vi "target.set.vi"(8 "error in (no error)":errorcluster, 10 "datasources.lvlib:target.lvclass":refnum<class "target.lvclass">, 11 "datasource in":refnum<class "datasource.lvclass">) -> (0 "error out":errorcluster, 3 "datasource out":refnum<class "datasource.lvclass">)   [LabVIEW 2020, in "datasources.lvlib" / "datasource.lvclass"]
uses:
  datasource.lvclass
  target/target.lvclass
  datasource.lvclass/datasource.ctl
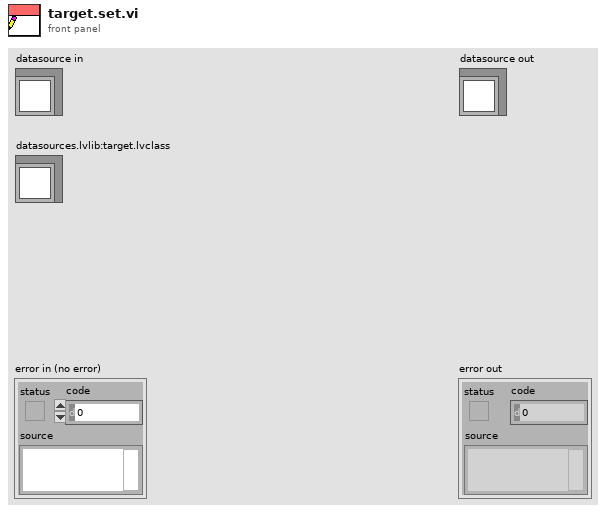
[diagram p1: front panel]
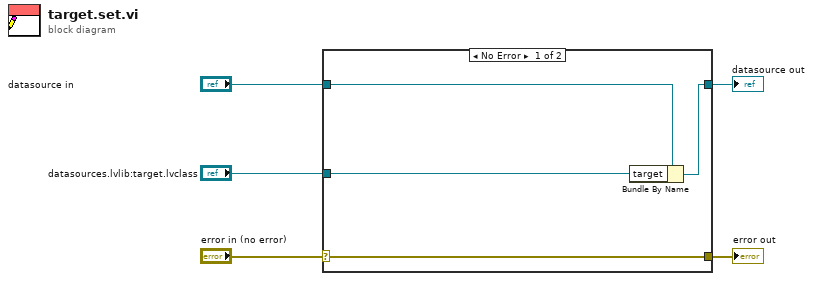
[diagram p0: block diagram]
diagram:
  n1 = case shown="No Error" "error in (no error)" {
    selector: "error in (no error)" -> [w9 w10]
    tunnel: [w9 w10] -> w4
    tunnel: [w7 w11] -> w2
    tunnel: "datasource in" -> [w8 w11]
    tunnel: "datasources.lvlib:target.lvclass" -> [w6 _]
    frame No Error {
      n2 = Bundle By Name(cluster=w8, "target"=w6) -> (w7:refnum<class "datasource.lvclass">)
    }
    frame Error {
    }
  }
  "error out" <- w4
  "datasource out" <- w2
